vi "Test Flatten.vi"() -> ()   [LabVIEW 2021]
uses:
  CIF_NIChn_Fifo_Power.lvclass
  ChannelCommon/typedef/FIFO Header.ctl
  ChannelCommon/ChannelCommon.lvlib
  ChannelCommon/typedef/Datatype Waveform.ctl
  ChannelCommon/typedef/TimeStamps.ctl
panel:
  in  "FIFO Timestamps":T1
  out "Data out":T2[](array[typedef])
  in  "Data In":T2[](array[typedef])=[{"measurement"=[0.0, 0.0, 0.0, 0.0, 0.0, 0.0, 0.0, 3.14], "dT"=0.01, "Timestamp"=498}, {"measurement"=[0.0, 0.0, 0.0, 0.0, 0.0, 0.0, 0.0, 9.8], "dT"=0.12, "Timestamp"=12345}]
  out "Header":T3={"Length"=52, "T0"=321, "T_Out"=123, "T_Tx"=1724093393726059437, "Ctr"=1, "ClockID"=0}
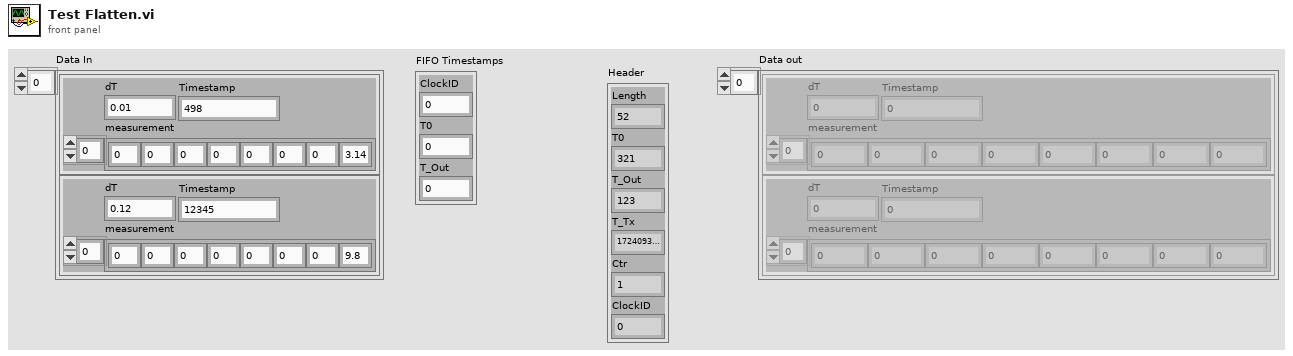
[diagram p1: front panel]
types:
  T1 = typedef "ChannelCommon.lvlib/TimeStamps.ctl" = cluster{"ClockID":u8, "T0":u64, "T_Out":u64}
  T2 = typedef "ChannelCommon.lvlib/Datatype Waveform.ctl" = cluster{"measurement":dbl[], "dT":dbl, "Timestamp":u64}
  T3 = typedef "ChannelCommon.lvlib/FIFO Header.ctl" = cluster{"Length":u64, "T0":u64, "T_Out":u64, "T_Tx":u64, "Ctr":u64, "ClockID":u8}
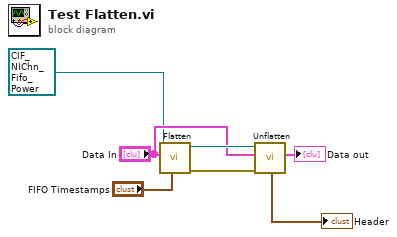
[diagram p0: block diagram]
diagram:
  n1 = call "Flatten.vi"("FIFO Timestamps"="FIFO Timestamps", "Data"="Data In", "CIFTag in"=refnum<class "CIF_NIChn_Fifo_Power.lvclass"> refnum ("CIF_NIChn_Fifo_Power.lvclass")) -> ("error out"=w6:errorcluster, "CIFTag out"=w7:refnum<class "CIF_NIChn_Fifo_Power.lvclass">)  [unwired: 6 in, 1 out]
  n2 = call "Unflatten.vi"("error in (no error)"=w6, "Data in"="Data In", "CIFFifoCAN in"=w7) -> ("Data out"=→"Data out":T2[], "Header"=→"Header":T3)  [unwired: 5 in, 2 out]
